vi "Create All Message Queues.vi"(8 "error in (no error)":errorcluster) -> (0 "error out":errorcluster, 3 "Message Queues out":T1)   [LabVIEW 2020, in "Message Queue.lvlib"]
doc: "This VI creates and initializes all the message queues for your application. If your application requires more than one message queue, right-click the \"Message Queues\" constant above and select Open Type Def. Add the new Message Queue(s) to the type definition, then initialize them in this VI."
uses:
  Message Queue.lvlib
  All Message Queues.ctl
  Message Cluster.ctl
  Enqueue Message (Single).vi
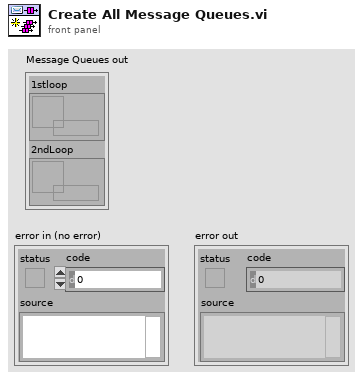
[diagram p1: front panel]
types:
  T1 = typedef "Message Queue.lvlib/All Message Queues.ctl" = cluster{"1stloop":refnum<queue>, "2ndLoop":refnum<queue>}
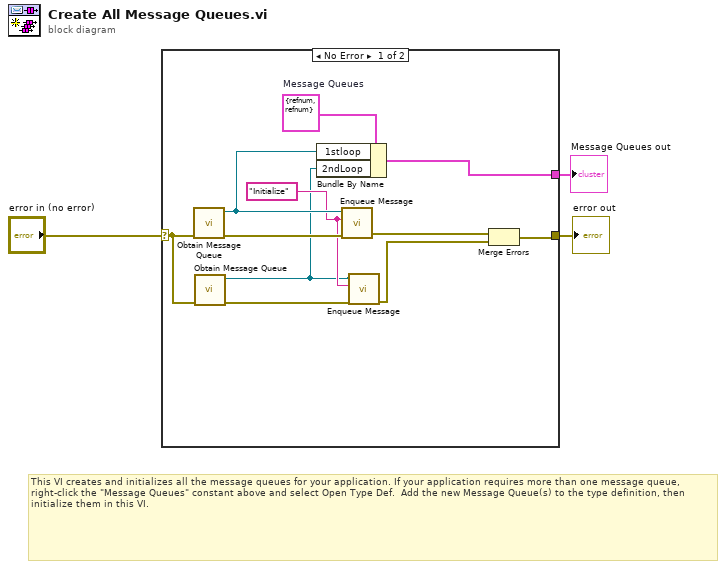
[diagram p0: block diagram]
diagram:
  # "This VI creates and initializes all the message queues for your application. If your application requires more than one message queue, right-click the \"Message Queues\" constant above and select Open Type Def.  Add the new Message Queue(s) to the type definition, then initialize them in this VI."
  n1 = case shown="No Error" "error in (no error)" {
    selector: "error in (no error)" -> [w10 w15]
    tunnel: [w5 w15] -> w3
    tunnel: [w13 _] -> w2
    frame No Error {
      w9 = "Initialize" ("Message")
      w14 = T1 {"1stloop"=refnum, "2ndLoop"=refnum}  # Message Queues
      n2 = call "Obtain Message Queue.vi"("error in (no error)"=w10) -> ("error out"=w12:errorcluster, "Message Queue"=w11:refnum<queue>)  [unwired: 9 in]
      n3 = call "Obtain Message Queue.vi"("error in (no error)"=w10) -> ("error out"=w7:errorcluster, "Message Queue"=w8:refnum<queue>)  [unwired: 9 in]
      n4 = Bundle By Name(cluster=w14, "1stloop"=w11, "2ndLoop"=w8) -> (w13:T1)
      n5 = call-poly "Enqueue Message.vi"("error in (no error)"=w12, "Message"=w9, "Message Queue"=w11) -> ("error out"=w4:errorcluster)  [unwired: 7 in, 1 out]
      n6 = call-poly "Enqueue Message.vi"("error in (no error)"=w7, "Message"=w9, "Message Queue"=w8) -> ("error out"=w6:errorcluster)  [unwired: 7 in, 1 out]
      n7 = Merge Errors(w4, w6) -> (w5:errorcluster)
    }
    frame Error {
    }
  }
  "Message Queues out" <- w2
  "error out" <- w3
